vi "Telescope Init.vi"(8 "error in (no error)":errorcluster, 9 "Settings":variant, 10 "Name":string, 11 "Telescope Simulator in":refnum<class "Telescope Simulator.lvclass">) -> (0 "error out":errorcluster, 1 "Connect Message":string, 2 "Channel List":refnum<class "HK Item.lvclass">[](array[class]), 3 "Telescope Simulator out":refnum<class "Telescope Simulator.lvclass">)   [LabVIEW 2024, in "Telescope Simulator.lvclass"]
uses:
  Telescope Simulator.lvclass
  hk-channel-class/hk-channel-class/HK Item/HK Item.lvclass
  Telescope Simulator cluster Settings.ctl
  Telescope enum Status.ctl
  Telescope Simulator.lvclass/Telescope Simulator.ctl
  Telescope.lvclass
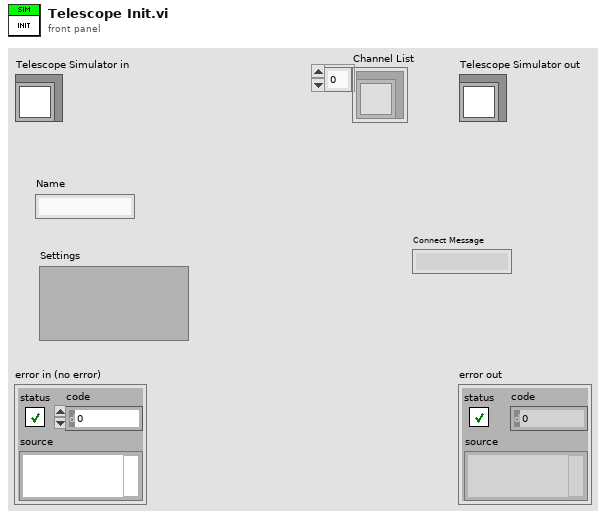
[diagram p1: front panel]
types:
  T1 = typedef "Telescope.lvclass/Telescope enum Status.ctl" = enum16{"Initializing", "Ready", "Moving", "Focusing", "Error"}
  T2 = typedef "Telescope Simulator cluster Settings.ctl" = cluster{"move rate":dbl}
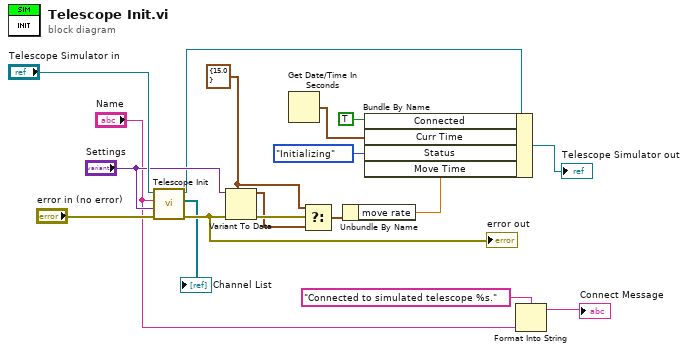
[diagram p0: block diagram]
diagram:
  w11 = T2 {"move rate"=15.0}
  n1 = call-parent "Telescope Init.vi"("error in (no error)"="error in (no error)", "Settings"="Settings", "Name"="Name", "Telescope in"="Telescope Simulator in") -> ("error out"=w8:errorcluster, "Channel List"=→"Channel List":refnum<class "HK Item.lvclass">[], "Telescope out"=w15:refnum<class "Telescope Simulator.lvclass">)  [unwired: 4 in, 1 out]
  "error out" <- w8
  n2 = Variant To Data(error in=w8, type=w11, Variant="Settings") -> (data=w12:T2, error out=w13:errorcluster)
  n3 = Get Date/Time In Seconds() -> (seconds since 1Jan1904=w6:timestamp)
  n4 = Select(t=w11, s=w13, f=w12) -> (s? t:f=w10:T2)
  n5 = Unbundle By Name(w10) -> ("move rate"=w9:dbl)
  n6 = Bundle By Name(cluster=w15, "Connected"=TRUE ("Telescope Status.Connected"), "Curr Time"=w6, "Status"=Telescope_enum_Status."Initializing" ("Telescope Status.Status"), "Move Time"=w9) -> (→"Telescope Simulator out":refnum<class "Telescope Simulator.lvclass">)
  n7 = Format Into String(format string="Connected to simulated telescope %s." ("Connect Message"), "Name") -> (resulting string=→"Connect Message":string)  [unwired: 2 in, 1 out]
